vi "SetCommand.vi"(7 "ButtonIndex(0..n)":i32, 8 "error in":errorcluster, 9 "OffCommand":refnum<class "Command.lvclass">, 10 "OnCommand":refnum<class "Command.lvclass">, 11 "reference in":refnum<class "RemoteControl.lvclass">) -> (0 "error out":errorcluster, 3 "reference out":refnum<class "RemoteControl.lvclass">)   [LabVIEW 2020, in "RemoteControl.lvclass"]
uses:
  RemoteControl.lvclass
  Command_class/Command.lvclass
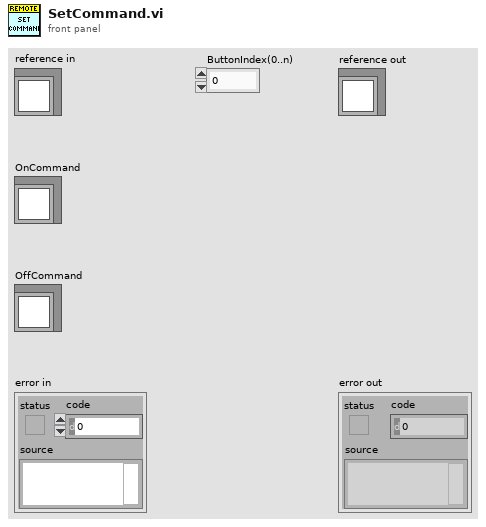
[diagram p1: front panel]
types:
  T1 = typedef "RemoteControl.lvclass/ObjectAttributes.ctl" = cluster{"OnCommands":refnum<class "Command.lvclass">[], "OffCommands":refnum<class "Command.lvclass">[], "UndoCommand":refnum<class "Command.lvclass">}
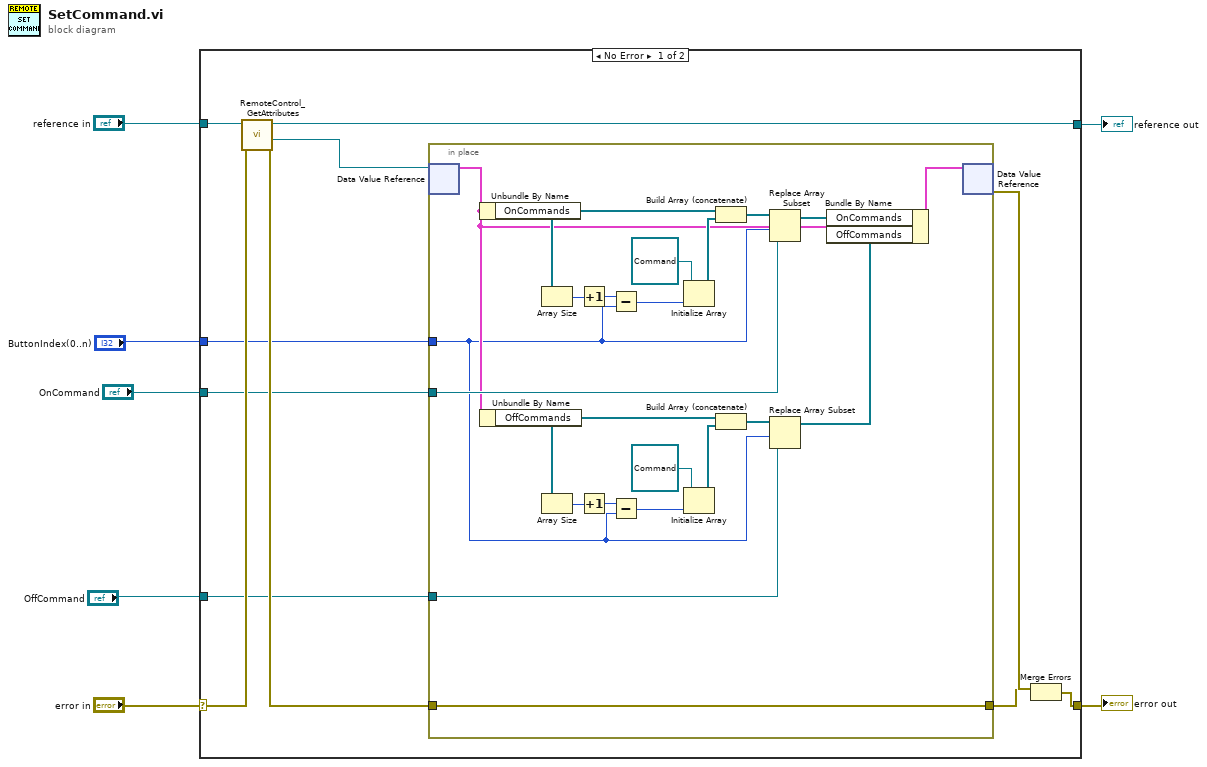
[diagram p0: block diagram]
diagram:
  n1 = case shown="No Error" "error in" {
    selector: "error in" -> [w18 w42]
    tunnel: [w16 w42] -> w6
    tunnel: [w12 w41] -> w4
    tunnel: "reference in" -> [w13 w41]
    tunnel: "ButtonIndex(0..n)" -> [w10 _]
    tunnel: "OnCommand" -> [w9 _]
    tunnel: "OffCommand" -> [w8 _]
    frame No Error {
      n2 = call "RemoteControl_GetAttributes.vi"("error in (no error)"=w18, "reference in"=w13) -> ("error out"=w15:errorcluster, "DataRef"=w11:refnum<data-value>, "reference out"=w12:refnum<class "RemoteControl.lvclass">)  [unwired: 6 in, 1 out]
      n3 = in-place {
        in-place-border: w15 -> [w40]
        in-place-border: [w40] -> w14
        in-place-border: w10 -> [w20]
        in-place-border: w9 -> [w30]
        in-place-border: w8 -> [w19]
        n4 = in-place-dvr #1(w11) -> (w22:T1)  [unwired: 1 out]
        n5 = Unbundle By Name(w22) -> ("OnCommands"=w34:refnum<class "Command.lvclass">[])
        n6 = Unbundle By Name(w22) -> ("OffCommands"=w27:refnum<class "Command.lvclass">[])
        n7 = Array Size(array=w34) -> (size(s)=w38:i32)
        n8 = Array Size(array=w27) -> (size(s)=w23:i32)
        n9 = Increment(x=w38) -> (x+1=w33:i32)
        n10 = Increment(x=w23) -> (x+1=w28:i32)
        n11 = Subtract(x=w33, y=w20) -> (x-y=w37:i32)
        n12 = Subtract(x=w28, y=w20) -> (x-y=w24:i32)
        n13 = Initialize Array(refnum<class "Command.lvclass"> refnum ("Command"), w37) -> (w35:refnum<class "Command.lvclass">[])
        n14 = Initialize Array(refnum<class "Command.lvclass"> refnum ("Command"), w24) -> (w26:refnum<class "Command.lvclass">[])
        n15 = Build Array (concatenate)(w34, w35) -> (w32:refnum<class "Command.lvclass">[])
        n16 = Build Array (concatenate)(w27, w26) -> (w29:refnum<class "Command.lvclass">[])
        n17 = Replace Array Subset(array=w32, new element=w30, index=w20) -> (w31:refnum<class "Command.lvclass">[])
        n18 = Replace Array Subset(array=w29, new element=w19, index=w20) -> (w21:refnum<class "Command.lvclass">[])
        n19 = Bundle By Name(cluster=w22, "OnCommands"=w31, "OffCommands"=w21) -> (w39:T1)
        n20 = in-place-dvr #1(w39) -> (w17:errorcluster)  [unwired: 1 out]
      }
      n21 = Merge Errors(w17, w14) -> (w16:errorcluster)
    }
    frame Error {
    }
  }
  "error out" <- w6
  "reference out" <- w4
